vi "Decode status bits.vi"(10 "Status bits":u16, 11 "F-70 parameters in in":T1 {"Last updated" format="%<%d/%m/%Y %H:%M:%S>T"; "State of operation" items=["Local Off", "Local On", "Remote Off", "Remote On", "Cold head Run", "Cold head pause", "Fault Off", "Oil Fault Off"]; "Return pressure (PSIG)" scale=0.0..200.0; "Water in Tmp (°C)" scale=0.0..100.0; "Water out Tmp (°C)" scale=0.0..100.0; "He discharge Tmp (°C)" scale=0.0..100.0}) -> (3 "F-70 parameters out":T1 {"Last updated" format="%<%d/%m/%Y %H:%M:%S>T"; "State of operation" items=["Local Off", "Local On", "Remote Off", "Remote On", "Cold head Run", "Cold head pause", "Fault Off", "Oil Fault Off"]; "Return pressure (PSIG)" scale=0.0..200.0; "Water in Tmp (°C)" scale=0.0..100.0; "Water out Tmp (°C)" scale=0.0..100.0; "He discharge Tmp (°C)" scale=0.0..100.0})   [LabVIEW 2021, in "F-70 driver.lvlib"]
uses:
  F-70 driver.lvlib
  public/F-70 parameters.ctl
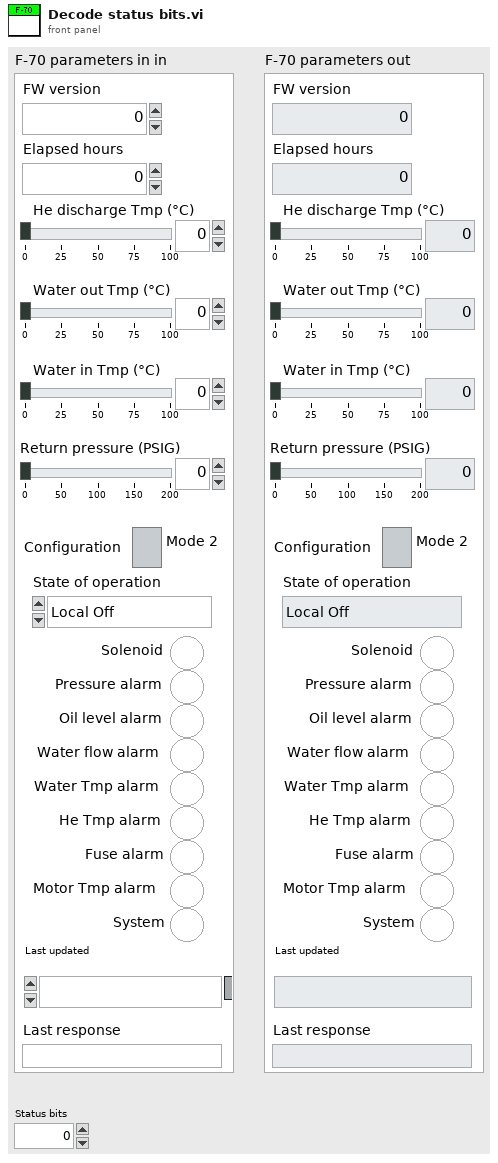
[diagram p1: front panel]
types:
  T1 = typedef "F-70 driver.lvlib/F-70 parameters.ctl" = cluster{"FW version":dbl, "Elapsed hours":dbl, "He discharge Tmp (°C)":dbl, "Water out Tmp (°C)":dbl, "Water in Tmp (°C)":dbl, "Return pressure (PSIG)":dbl, "Configuration":bool, "State of operation":u16, "Solenoid":bool, "Pressure alarm":bool, "Oil level alarm":bool, "Water flow alarm":bool, "Water Tmp alarm":bool, "He Tmp alarm":bool, "Fuse alarm":bool, "Motor Tmp alarm":bool, "System":bool, "Last updated":timestamp, "Last response":string}
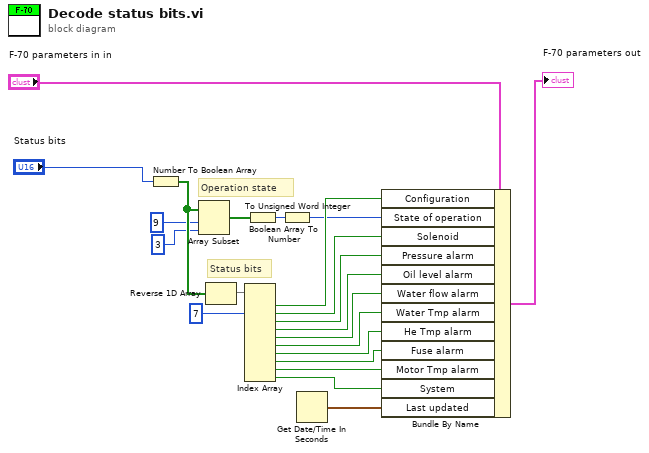
[diagram p0: block diagram]
diagram:
  # "Status bits"
  # "Operation state"
  n1 = Number To Boolean Array(number="Status bits") -> (Boolean array=w8:bool[])
  n2 = Array Subset(array=w8, index=9, length=3) -> (w6:bool[])
  n3 = Reverse 1D Array(array=w8) -> (reversed array=w11:bool[])
  n4 = Index Array(array=w11, index #2=7 ("index")) -> (element #1=w12:bool, element #2=w14:bool, element #3=w15:bool, element #4=w16:bool, element #5=w17:bool, element #6=w18:bool, element #7=w19:bool, element #8=w20:bool, element #9=w21:bool, element #10=w22:bool)  [unwired: 9 in]
  n5 = Boolean Array To Number(Boolean array=w6) -> (number=w9:u32)
  n6 = To Unsigned Word Integer(number=w9) -> (unsigned 16bit integer=w10:u16)
  n7 = Get Date/Time In Seconds() -> (seconds since 1Jan1904=w3:timestamp)
  n8 = Bundle By Name(cluster="F-70 parameters in in", "Configuration"=w12, "State of operation"=w10, "Solenoid"=w14, "Pressure alarm"=w15, "Oil level alarm"=w16, "Water flow alarm"=w17, "Water Tmp alarm"=w18, "He Tmp alarm"=w19, "Fuse alarm"=w20, "Motor Tmp alarm"=w21, "System"=w22, "Last updated"=w3) -> (→"F-70 parameters out":T1)
